vi "WPI_DashboardRename Videos.vi"(10 "Path":path, 11 "Log Name":string) -> ()   [LabVIEW 2019]
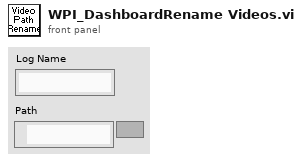
[diagram p1: front panel]
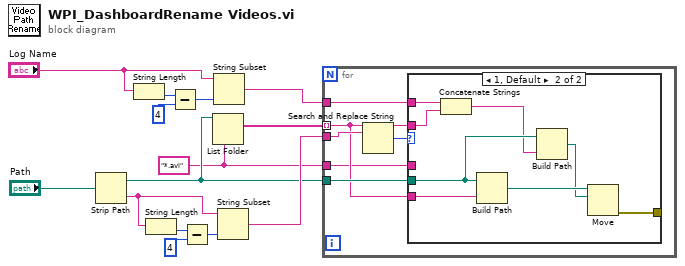
[diagram p0: block diagram]
diagram:
  w2 = "*.avi"
  n1 = Strip Path(path="Path") -> (stripped path=w8:path, name=w12:string)
  n2 = String Length(string="Log Name") -> (length=w6:i32)
  n3 = String Length(string=w12) -> (length=w13:i32)
  n4 = Subtract(x=w6, y=4) -> (x-y=w7:i32)
  n5 = Subtract(x=w13, y=4) -> (x-y=w11:i32)
  n6 = List Folder(path=w8, pattern=w2) -> (filenames=w9:string[])  [unwired: 2 in, 3 out]
  n7 = String Subset(string="Log Name", length (rest)=w7) -> (substring=w3:string)  [unwired: 1 in]
  n8 = String Subset(string=w12, length (rest)=w11) -> (substring=w10:string)  [unwired: 1 in]
  n9 = for {
    tunnel: w9 -> [w18] mode=indexing
    tunnel: w10 -> [w21]
    tunnel: w8 -> [w19]
    tunnel: w3 -> [w16]
    tunnel: w2 -> [w15]
    n10 = Search and Replace String(input string=w18, search string=w21) -> (result string=w17:string, number of replacements=w20:i32)  [unwired: 6 in, 2 out]
    n11 = case shown="1, Default" w20 {
      tunnel: w19 -> [_ w27]
      tunnel: w18 -> [_ w29]
      tunnel: w17 -> [_ w25]
      tunnel: w16 -> [_ w24]
      tunnel: w15 -> [_ _]
      tunnel: [_ w22] -> _
      frame 0 {
      }
      frame 1, Default {
        n12 = Concatenate Strings(w24, w25) -> (w23:string)
        n13 = Build Path(base path=w27, name or relative path=w29) -> (appended path=w28:path)
        n14 = Build Path(base path=w27, name or relative path=w23) -> (appended path=w26:path)
        n15 = Move(source path=w28, 10:w26) -> (error out=w22:errorcluster)  [unwired: 3 in, 2 out]
      }
    }
  }
